vi "AeroQuadUploader32.vi"(10 "URL":string="http://aq32.aeroquad.com", 11 "Com Port":refnum<visa-resource-name>) -> (3 "Com Port Out":refnum<visa-resource-name>)   [LabVIEW 2010]
uses:
  <vilib>/httpClient/LabVIEWHTTPClient.lvlib
panel:
  in  "WebBrowser":refnum<k7>(container)
  out "Status":string="AeroQuad 32 Uploader"
  in  "Restart":bool
  in  "Done":bool
  in  "Upload":bool
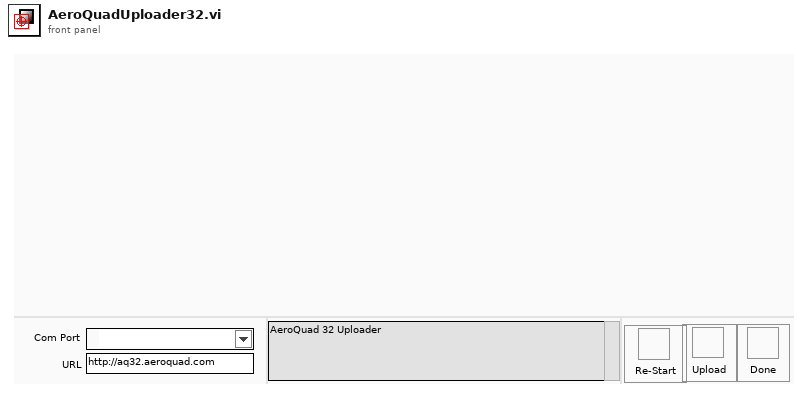
[diagram p1: front panel]
types:
  T1 = cluster{"Connected":bool, "WebBrowser":refnum<k7>, "WorkingFolder":path, "HTML":string, "Counter":i32}
  T2 = enum32{"invalid app kind", "Development System", "Run Time System", "Student Edition", "Embedded LabVIEW", "Evaluation", "Custom"}
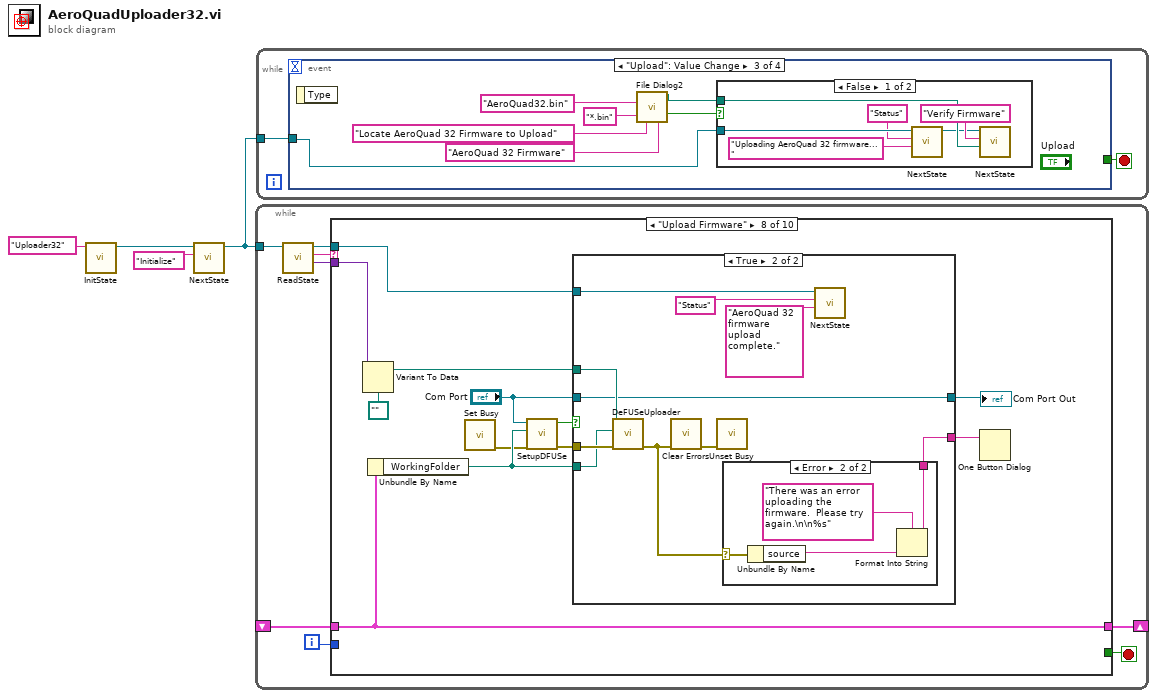
[diagram p0: block diagram]
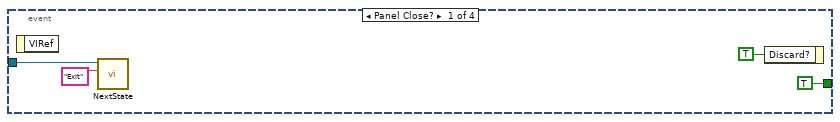
[diagram p2: hidden frame]
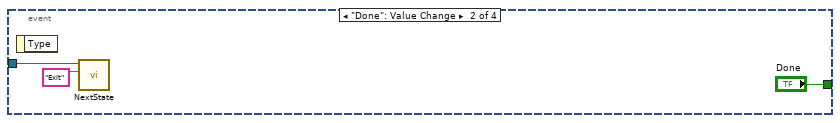
[diagram p3: hidden frame]
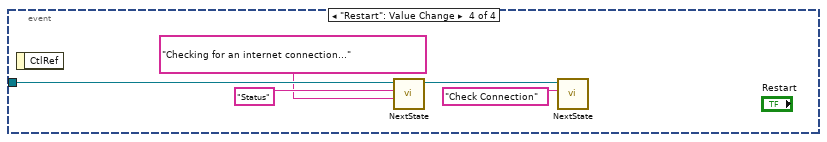
[diagram p5: hidden frame]
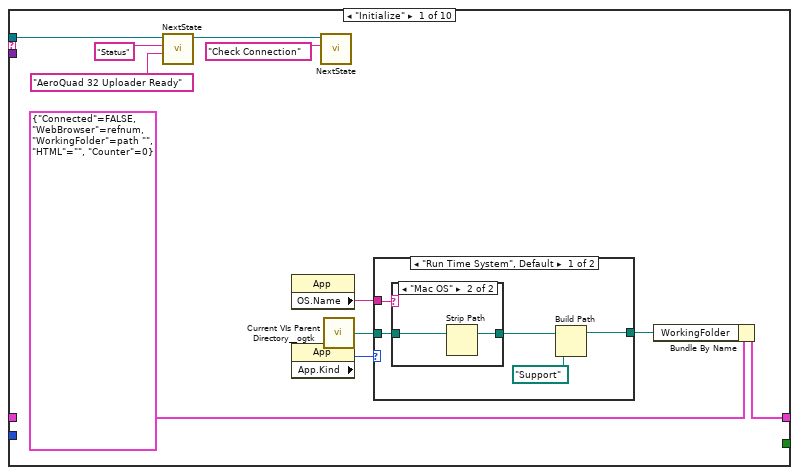
[diagram p6: hidden frame]
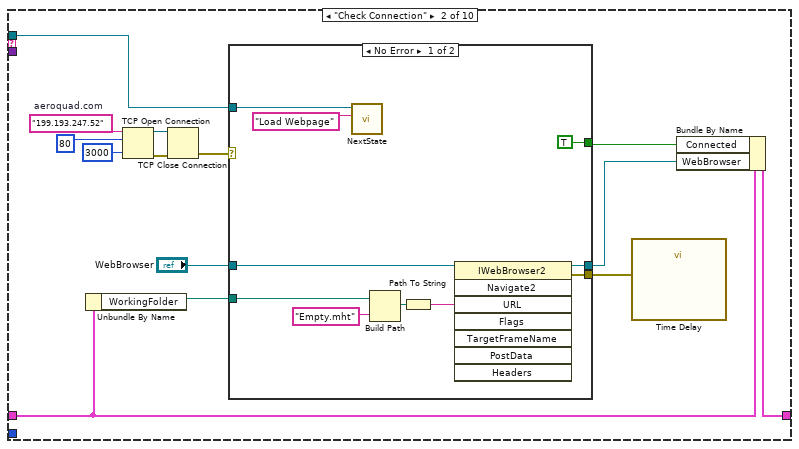
[diagram p9: hidden frame]
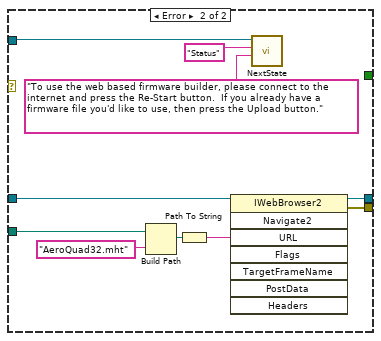
[diagram p10: hidden frame]
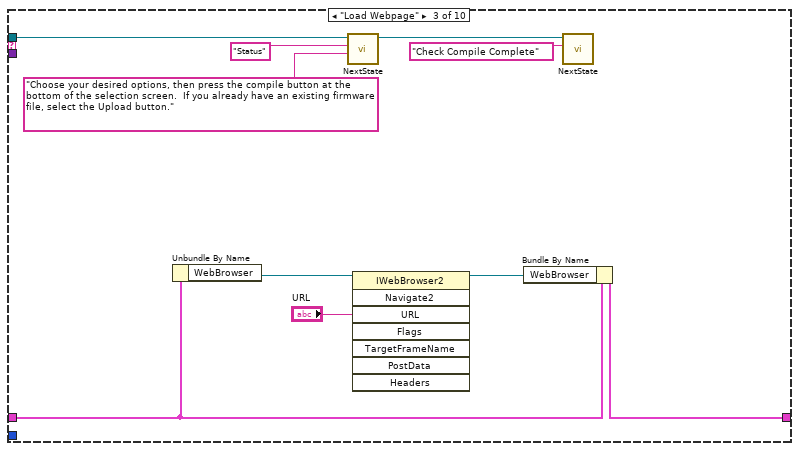
[diagram p11: hidden frame]
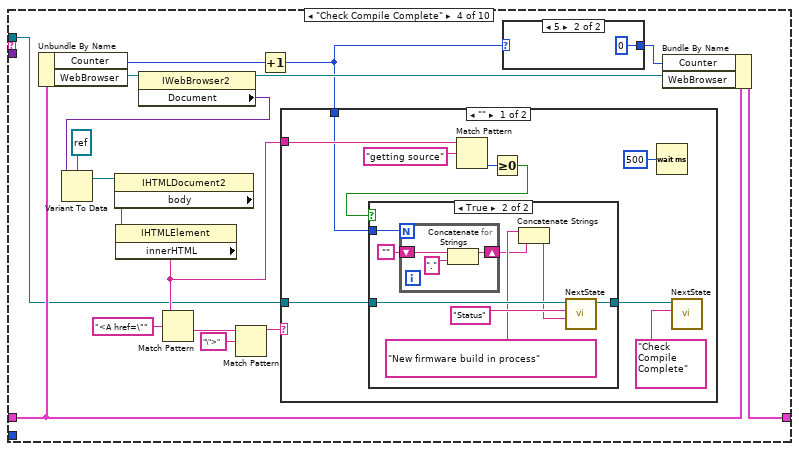
[diagram p12: hidden frame]
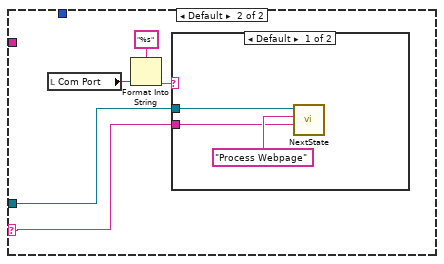
[diagram p15: hidden frame]
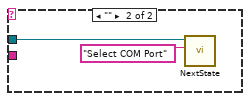
[diagram p16: hidden frame]
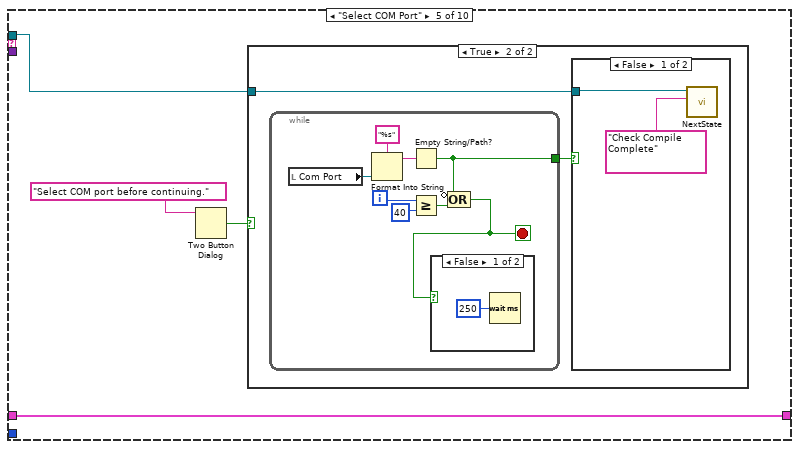
[diagram p17: hidden frame]
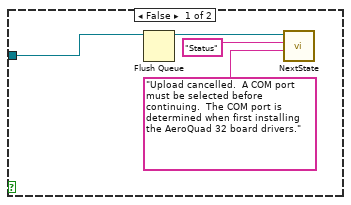
[diagram p18: hidden frame]
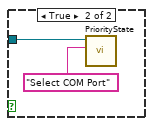
[diagram p19: hidden frame]
diagram:
  n1 = call "InitState.vi"("Name"="Uploader32") -> ("Queue Out"=w1:refnum<queue>)  [unwired: 8 in, 1 out]
  n2 = call "NextState.vi"("State"="Initialize", "Queue In"=w1) -> ("Queue Out"=w2:refnum<queue>)  [unwired: 8 in, 1 out]
  n3 = while {
    tunnel: w2 -> [w12]
    shift-right: [w7] -> _
    shift-left: _ -> [w6]
    i -> [w5]
    stop <- w8 stop-if-true
    n4 = call "ReadState.vi"("Queue In"=w12) -> ("Data"=w10:variant, "State"=w11:string, "Queue Out"=w9:refnum<queue>)  [unwired: 7 in, 1 out]
    n5 = case shown="\"Upload Firmware\"" w11 {
      selector: w11 -> [_ _ _ _ _ w162 _ _ w232 _]
      tunnel: w10 -> [_ _ _ _ _ w163 w186 w204 w233 _]
      tunnel: w9 -> [w13 w37 w72 w77 w127 w161 w184 w197 _ w234]
      tunnel: [_ _ _ _ _ _ _ _ _ TRUE] -> w8
      tunnel: [w18 w41 w75 w87 w130 w154 w179 w208 w230 w235] -> w7
      tunnel: w6 -> [_ w38 w68 w88 w130 w154 w179 w208 w230 w235]
      tunnel: w5 -> [_ _ _ _ _ _ _ _ _ _]
      frame "Initialize" {
        n6 = call "NextState.vi"("Data"="AeroQuad 32 Uploader Ready" ("State"), "State"="Status", "Queue In"=w13) -> ("Queue Out"=w14:refnum<queue>)  [unwired: 7 in, 1 out]
        n7 = property class="App"() -> ("OS.Name"=w20:string)  [unwired: 2 in, 2 out]
        n8 = property class="App"() -> ("App.Kind"=w22:T2)  [unwired: 2 in, 2 out]
        n9 = call "NextState.vi"("State"="Check Connection", "Queue In"=w14) -> ()  [unwired: 8 in, 2 out]
        n10 = call <userlib>:"Current VIs Parent Directory__ogtk.vi"() -> ("Parent Directory (+ Relative)"=w21:path)  [unwired: 5 in]
        n11 = case shown="\"Run Time System\", Default" w22 {
          tunnel: [w24 w32] -> w17
          tunnel: w21 -> [w27 w32]
          tunnel: w20 -> [w25 _]
          frame "Run Time System", Default {
            n12 = case shown="\"Mac OS\"" w25 {
              tunnel: [w29 w31] -> w28
              tunnel: w27 -> [w29 w30]
              frame Default {
              }
              frame "Mac OS" {
                n13 = Strip Path(path=w30) -> (stripped path=w31:path)  [unwired: 1 out]
              }
            }
            n14 = Build Path(base path=w28, name or relative path=path "Support") -> (appended path=w24:path)
          }
          frame "Development System" {
          }
        }
        n15 = Bundle By Name(cluster=T1 {"Connected"=FALSE, "WebBrowser"=refnum, "WorkingFolder"=path "", "HTML"="", "Counter"=0}, "WorkingFolder"=w17) -> (w18:T1)
      }
      frame "Check Connection" {
        w46 = "199.193.247.52"  # aeroquad.com
        n16 = Unbundle By Name(w38) -> ("WorkingFolder"=w36:path)
        n17 = TCP Open Connection(address=w46, remote port or service name=u16 80, timeout ms (60000)=3000) -> (connection ID=w42:refnum<k5>, error out=w43:errorcluster)  [unwired: 2 in]
        n18 = TCP Close Connection(connection ID=w42, error in (no error)=w43) -> (error out=w39:errorcluster)  [unwired: 1 in, 1 out]
        n19 = case shown="No Error" w39 {
          tunnel: w37 -> [w56 w66]
          tunnel: [TRUE _] -> w40
          tunnel: "WebBrowser" -> [w50 w60]
          tunnel: w36 -> [w49 w59]
          tunnel: [w48 w58] -> w35
          tunnel: [w47 w57] -> w34
          frame No Error {
            n20 = call "NextState.vi"("State"="Load Webpage", "Queue In"=w56) -> ()  [unwired: 8 in, 2 out]
            n21 = Build Path(base path=w49, name or relative path="Empty.mht") -> (appended path=w53:path)
            n22 = Path To String(path=w53) -> (string=w52:string)
            n23 = invoke class="IWebBrowser2" method="Navigate2"(reference=w50, "URL"=w52) -> (reference out=w48:refnum<k7>, error out=w47:errorcluster)  [unwired: 6 in, 6 out]
          }
          frame Error {
            n24 = Build Path(base path=w59, name or relative path="AeroQuad32.mht") -> (appended path=w63:path)
            n25 = Path To String(path=w63) -> (string=w62:string)
            n26 = invoke class="IWebBrowser2" method="Navigate2"(reference=w60, "URL"=w62) -> (reference out=w58:refnum<k7>, error out=w57:errorcluster)  [unwired: 6 in, 6 out]
            n27 = call "NextState.vi"("Data"="To use the web based firmware builder, please connect to the internet and press the Re-Start button.  If you already have a firmware file you'd like to use, then press the Upload button." ("State"), "State"="Status", "Queue In"=w66) -> ()  [unwired: 7 in, 2 out]
          }
        }
        n28 = call "Time Delay"("error in (no error)"=w34) -> ()  [unwired: 10 in, 1 out]
        n29 = Bundle By Name(cluster=w38, "Connected"=w40, "WebBrowser"=w35) -> (w41:T1)
      }
      frame "Load Webpage" {
        n30 = Unbundle By Name(w68) -> ("WebBrowser"=w67:refnum<k7>)
        n31 = call "NextState.vi"("Data"="Choose your desired options, then press the compile button at the bottom of the selection screen.  If you already have an existing firmware file, select the Upload button." ("State"), "State"="Status", "Queue In"=w72) -> ("Queue Out"=w71:refnum<queue>)  [unwired: 7 in, 1 out]
        n32 = invoke class="IWebBrowser2" method="Navigate2"(reference=w67, "URL"="URL") -> (reference out=w74:refnum<k7>)  [unwired: 6 in, 7 out]
        n33 = Bundle By Name(cluster=w68, "WebBrowser"=w74) -> (w75:T1)
        n34 = call "NextState.vi"("State"="Check Compile Complete", "Queue In"=w71) -> ()  [unwired: 8 in, 2 out]
      }
      frame "Check Compile Complete" {
        n35 = Unbundle By Name(w88) -> ("Counter"=w80:i32, "WebBrowser"=w92:refnum<k7>)
        n36 = property class="IWebBrowser2"(reference=w92) -> (reference out=w89:refnum<k7>, "Document"=w91:variant)  [unwired: 1 in, 1 out]
        n37 = Variant To Data(Variant=w91, type=refnum<k7> refnum ("WebBrowser")) -> (data=w82:refnum<k7>)  [unwired: 1 in, 1 out]
        n38 = property class="IHTMLDocument2"(reference=w82) -> ("body"=w90:refnum<k7>)  [unwired: 1 in, 2 out]
        n39 = property class="IHTMLElement"(reference=w90) -> ("innerHTML"=w81:string)  [unwired: 1 in, 2 out]
        n40 = Match Pattern(string=w81, regular expression="<A href=\"") -> (after substring=w85:string)  [unwired: 1 in, 3 out]
        n41 = Match Pattern(string=w85, regular expression="\">") -> (before substring=w83:string)  [unwired: 1 in, 3 out]
        n42 = Increment(x=w80) -> (x+1=w79:i32)
        n43 = case shown="\"\"" w83 {
          selector: w83 -> [_ w117]
          tunnel: w77 -> [w96 w118]
          tunnel: w81 -> [w102 _]
          tunnel: w79 -> [w97 _]
          frame "" {
            n44 = Match Pattern(string=w102, regular expression="getting source") -> (offset past match=w100:i32)  [unwired: 1 in, 3 out]
            n45 = Greater Or Equal To 0?(x=w100) -> (x >= 0?=w99:bool)
            n46 = case shown="True" w99 {
              tunnel: [w105 w113] -> w98
              tunnel: w96 -> [w105 w112]
              tunnel: w97 -> [_ w106]
              frame False {
              }
              frame True {
                n47 = for {
                  N: w106 -> [_]
                  shift-right: [w114] -> w108
                  shift-left: "" -> [w116]
                  n48 = Concatenate Strings(w116, ".") -> (w114:string)
                }
                n49 = Concatenate Strings("New firmware build in process" ("State"), w108) -> (w109:string)
                n50 = call "NextState.vi"("Data"=w109, "State"="Status", "Queue In"=w112) -> ("Queue Out"=w113:refnum<queue>)  [unwired: 7 in, 1 out]
              }
            }
            n51 = Wait (ms)(milliseconds to wait=u32 500) -> ()  [unwired: 1 out]
            n52 = call "NextState.vi"("State"="Check Compile Complete", "Queue In"=w98) -> ()  [unwired: 8 in, 2 out]
          }
          frame Default {
            n53 = local read "Com Port"() -> (w119:refnum<visa-resource-name>)
            n54 = Format Into String(format string="%s", w119) -> (resulting string=w121:string)  [unwired: 2 in, 1 out]
            n55 = case shown="Default" w121 {
              tunnel: w118 -> [w123 w125]
              tunnel: w117 -> [w122 _]
              frame Default {
                n56 = call "NextState.vi"("Data"=w122, "State"="Process Webpage", "Queue In"=w123) -> ()  [unwired: 7 in, 2 out]
              }
              frame "" {
                n57 = call "NextState.vi"("State"="Select COM Port", "Queue In"=w125) -> ()  [unwired: 8 in, 2 out]
              }
            }
          }
        }
        n58 = case shown="5" w79 {
          selector: w79 -> [w94 _]
          tunnel: [w94 0] -> w78
          frame Default {
          }
          frame 5 {
          }
        }
        n59 = Bundle By Name(cluster=w88, "Counter"=w78, "WebBrowser"=w89) -> (w87:T1)
      }
      frame "Select COM Port" {
        n60 = Two Button Dialog(message="Select COM port before continuing.") -> (T button?=w128:bool)  [unwired: 2 in]
        n61 = case shown="True" w128 {
          tunnel: w127 -> [w134 w136]
          frame False {
            n62 = Flush Queue(queue=w134) -> (queue out=w133:refnum<queue>)  [unwired: 1 in, 2 out]
            n63 = call "NextState.vi"("Data"="Upload cancelled.  A COM port must be selected before continuing.  The COM port is determined when first installing the AeroQuad 32 board drivers." ("State"), "State"="Status", "Queue In"=w133) -> ()  [unwired: 7 in, 2 out]
          }
          frame True {
            n64 = while {
              tunnel: [w141] -> w135
              i -> [w145]
              stop <- w142 stop-if-true
              n65 = local read "Com Port"() -> (w147:refnum<visa-resource-name>)
              n66 = Format Into String(format string="%s", w147) -> (resulting string=w146:string)  [unwired: 2 in, 1 out]
              n67 = Empty String/Path?(string/path=w146) -> (empty?=w141:bool)
              n68 = Greater Or Equal?(x=w145, y=40) -> (x >= y?=w143:bool)
              n69 = Compound Arithmetic op=OR(invert w141, w143) -> (w142:bool)
              n70 = case shown="False" w142 {
                frame False {
                  n71 = Wait (ms)(milliseconds to wait=u32 250) -> ()  [unwired: 1 out]
                }
                frame True {
                }
              }
            }
            n72 = case shown="False" w135 {
              tunnel: w136 -> [w138 w140]
              frame False {
                n73 = call "NextState.vi"("State"="Check Compile Complete", "Queue In"=w138) -> ()  [unwired: 8 in, 2 out]
              }
              frame True {
                n74 = call "PriorityState.vi"("State"="Select COM Port", "Queue In"=w140) -> ()  [unwired: 8 in, 2 out]
              }
            }
          }
        }
      }
      frame "Process Webpage" {
        n75 = Variant To Data(Variant=w163, type=w162) -> (data=w152:string)  [unwired: 1 in, 1 out]
        n76 = Concatenate Strings("http://kari.hautio.net" ("string"), w152) -> (w150:string)
        n77 = Flush Queue(queue=w161) -> (queue out=w155:refnum<queue>)  [unwired: 1 in, 2 out]
        n78 = call "File Dialog"("prompt"="Select Location to Save AeroQuad 32 Firmware", "default name"="AeroQuad32.bin", "pattern (all files)"="*.bin", "pattern label"="AeroQuad 32 Firmware") -> ("selected path"=w151:path, "cancelled"=w160:bool)  [unwired: 8 in, 2 out]
        n79 = case shown="True" w160 {
          tunnel: w150 -> [w167 _]
          tunnel: w151 -> [w166 _]
          tunnel: w155 -> [w168 w176]
          frame False {
            n80 = Delete(path (use dialog)=w166, confirm (F)=TRUE) -> (cancelled=w165:bool)  [unwired: 3 in, 2 out]
            n81 = case shown="True" w165 {
              tunnel: w168 -> [w172 w175]
              tunnel: w167 -> [w171 _]
              tunnel: w166 -> [w169 _]
              frame False {
                n82 = call <vilib>:"GET.vi"("output file"=w169, "URL"=w171) -> ()  [unwired: 10 in, 4 out]
                n83 = call "NextState.vi"("Data"=w169, "State"="Verify Firmware", "Queue In"=w172) -> ()  [unwired: 7 in, 2 out]
              }
              frame True {
                n84 = call "NextState.vi"("Data"="Upload cancelled." ("State"), "State"="Status", "Queue In"=w175) -> ()  [unwired: 7 in, 2 out]
              }
            }
          }
          frame True {
            n85 = call "NextState.vi"("Data"="Upload cancelled." ("State"), "State"="Status", "Queue In"=w176) -> ()  [unwired: 7 in, 2 out]
          }
        }
      }
      frame "Verify Firmware" {
        n86 = Variant To Data(Variant=w186, type=path "" ("selected path")) -> (data=w181:path)  [unwired: 1 in, 1 out]
        n87 = File/Directory Info(path=w181) -> (size=w180:i64)  [unwired: 1 in, 6 out]
        n88 = Greater Or Equal?(x=w180, y=i64 2000) -> (x >= y?=w182:bool)
        n89 = case shown="True" w182 {
          tunnel: w184 -> [w188 w192]
          tunnel: w181 -> [_ w195]
          frame False {
            n90 = Flush Queue(queue=w188) -> (queue out=w187:refnum<queue>)  [unwired: 1 in, 2 out]
            n91 = call "NextState.vi"("Data"="Invalid AeroQuad 32 firmware size detected (<2k).  Select or build another firmware binary and try again.  To build another binary select the Re-Start button.  Upload cancelled.", "State"="Status", "Queue In"=w187) -> ()  [unwired: 7 in, 2 out]
          }
          frame True {
            n92 = call "NextState.vi"("Data"="Valid firmware file verified.  Please wait, uploading firmware to the AeroQuad 32 board.  This may take a few minutes..." ("State"), "State"="Status", "Queue In"=w192) -> ("Queue Out"=w191:refnum<queue>)  [unwired: 7 in, 1 out]
            n93 = call "NextState.vi"("Data"=w195, "State"="Upload Firmware", "Queue In"=w191) -> ()  [unwired: 7 in, 2 out]
          }
        }
      }
      frame "Upload Firmware" {
        n94 = Variant To Data(Variant=w204, type=path "") -> (data=w202:path)  [unwired: 1 in, 1 out]
        n95 = Unbundle By Name(w208) -> ("WorkingFolder"=w201:path)
        n96 = call <vilib>:"Set Busy.vi"() -> ("error out"=w198:errorcluster)  [unwired: 10 in, 1 out]
        n97 = call "SetupDFUSe.vi"("Error In"=w198, "Working Directory"=w201, "Serial Port"="Com Port") -> ("Error"=w205:errorcluster, "Success"=w207:bool)  [unwired: 6 in]
        n98 = case shown="True" w207 {
          tunnel: "Com Port" -> [_ w218]
          tunnel: w205 -> [w210 w224]
          tunnel: w202 -> [_ w223]
          tunnel: w201 -> [_ w222]
          tunnel: ["Verify AeroQuad connected correctly and the correct COM port is selected. Unable to place the AeroQuad 32 board into programming mode.  If you have continued problems, try re-connecting the board and re-starting the uploader." ("message") w215] -> w200
          tunnel: w197 -> [w211 w219]
          tunnel: [_ w218] -> w199
          frame False {
            n99 = call <vilib>:"Clear Errors.vi"("error in (no error)"=w210) -> ("error out"=w209:errorcluster)  [unwired: 6 in]
            n100 = call <vilib>:"Unset Busy.vi"("error in (no error)"=w209) -> ()  [unwired: 10 in, 1 out]
            n101 = call "NextState.vi"("Data"="Press Re-Start to create a new firmware file or Upload to load an existing file." ("State"), "State"="Status", "Queue In"=w211) -> ()  [unwired: 7 in, 2 out]
          }
          frame True {
            n102 = call "DeFUSeUploader.vi"("Error In"=w224, "DFU-Util Working Directory"=w222, "Binary Filename"=w223) -> ("Error Out"=w216:errorcluster)  [unwired: 8 in]
            n103 = call <vilib>:"Clear Errors.vi"("error in (no error)"=w216) -> ("error out"=w217:errorcluster)  [unwired: 6 in]
            n104 = call <vilib>:"Unset Busy.vi"("error in (no error)"=w217) -> ()  [unwired: 10 in, 1 out]
            n105 = case shown="Error" w216 {
              selector: w216 -> [_ w227]
              tunnel: ["AeroQuad 32 firmware successfully uploaded." ("message") w228] -> w215
              frame No Error {
              }
              frame Error {
                n106 = Unbundle By Name(w227) -> ("source"=w226:string)
                n107 = Format Into String(format string="There was an error uploading the firmware.  Please try again.\n\n%s" ("message"), w226) -> (resulting string=w228:string)  [unwired: 2 in, 1 out]
              }
            }
            n108 = call "NextState.vi"("Data"="AeroQuad 32 firmware upload complete." ("State"), "State"="Status", "Queue In"=w219) -> ()  [unwired: 7 in, 2 out]
          }
        }
        "Com Port Out" <- w199
        n109 = One Button Dialog(message=w200) -> ()  [unwired: 1 in, 1 out]
      }
      frame "Status" {
        n110 = Variant To Data(Variant=w233, type=w232) -> (data=→"Status":string)  [unwired: 1 in, 1 out]
      }
      frame "Exit", Default {
        n111 = Release Queue(queue=w234) -> ()  [unwired: 2 in, 3 out]
      }
    }
  }
  n112 = while {
    tunnel: w2 -> [w237]
    stop <- w238 stop-if-true
    n113 = event shown="[2] \"Upload\": Value Change" {
      selector: _ -> [_ _ _ _]
      dyn-events: _ -> [_ _ _ _]
      timeout: _ -> [_ _ _ _]
      tunnel: [TRUE ("Done") "Done" _ _] -> w238
      tunnel: w237 -> [w240 w244 w248 w260]
      event Panel Close? {
        n114 = event-data() -> ()  [unwired: 1 in, 1 out]
        n115 = call "NextState.vi"("State"="Exit", "Queue In"=w240) -> ()  [unwired: 8 in, 2 out]
        n116 = event-data("Discard?"=TRUE) -> ()  [unwired: 1 in, 1 out]
      }
      event "Done": Value Change {
        n117 = event-data() -> ()  [unwired: 1 in, 1 out]
        n118 = call "NextState.vi"("State"="Exit", "Queue In"=w244) -> ()  [unwired: 8 in, 2 out]
      }
      event "Upload": Value Change {
        n119 = event-data() -> ()  [unwired: 1 in, 1 out]
        n120 = call "File Dialog2"("prompt"="Locate AeroQuad 32 Firmware to Upload", "default name"="AeroQuad32.bin", "pattern (all files)"="*.bin", "pattern label"="AeroQuad 32 Firmware") -> ("selected path"=w246:path, "cancelled"=w247:bool)  [unwired: 8 in, 2 out]
        n121 = case shown="False" w247 {
          tunnel: w248 -> [w255 _]
          tunnel: w246 -> [w257 _]
          frame False {
            n122 = call "NextState.vi"("Data"="Uploading AeroQuad 32 firmware..." ("State"), "State"="Status", "Queue In"=w255) -> ("Queue Out"=w256:refnum<queue>)  [unwired: 7 in, 1 out]
            n123 = call "NextState.vi"("Data"=w257, "State"="Verify Firmware", "Queue In"=w256) -> ()  [unwired: 7 in, 2 out]
          }
          frame True {
          }
        }
      }
      event "Restart": Value Change {
        n124 = event-data() -> ()  [unwired: 1 in, 1 out]
        n125 = call "NextState.vi"("Data"="Checking for an internet connection..." ("State"), "State"="Status", "Queue In"=w260) -> ("Queue Out"=w261:refnum<queue>)  [unwired: 7 in, 1 out]
        n126 = call "NextState.vi"("State"="Check Connection", "Queue In"=w261) -> ()  [unwired: 8 in, 2 out]
      }
    }
  }
